vi "color code.vi"(11 "Ch 1":dbl) -> (3 "Array":cluster{u32, u32}[](array[cluster]))   [LabVIEW 2016, in "CML UI.lvlib"]
uses:
  CML UI.lvlib
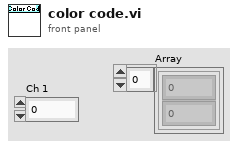
[diagram p1: front panel]
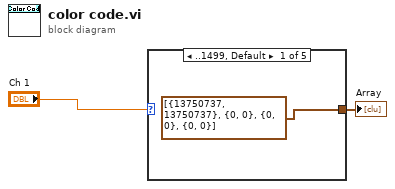
[diagram p0: block diagram]
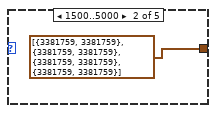
[diagram p2: hidden frame]
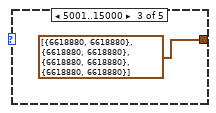
[diagram p3: hidden frame]
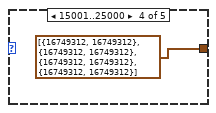
[diagram p4: hidden frame]
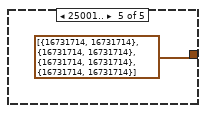
[diagram p5: hidden frame]
diagram:
  n1 = case shown="..1499, Default" "Ch 1" {
    tunnel: [cluster{u32, u32}[] [{13750737, 13750737}, {0, 0}, {0, 0}, {0, 0}] cluster{u32, u32}[] [{3381759, 3381759}, {3381759, 3381759}, {3381759, 3381759}, {3381759, 3381759}] cluster{u32, u32}[] [{6618880, 6618880}, {6618880, 6618880}, {6618880, 6618880}, {6618880, 6618880}] cluster{u32, u32}[] [{16749312, 16749312}, {16749312, 16749312}, {16749312, 16749312}, {16749312, 16749312}] cluster{u32, u32}[] [{16731714, 16731714}, {16731714, 16731714}, {16731714, 16731714}, {16731714, 16731714}]] -> w1
    frame ..1499, Default {
    }
    frame 1500..5000 {
    }
    frame 5001..15000 {
    }
    frame 15001..25000 {
    }
    frame 25001.. {
    }
  }
  "Array" <- w1
